vi "Get Head.vi"(11 "Snake in":refnum<class "Snake.lvclass">) -> (2 "Coordinates":T1)   [LabVIEW 2020, in "Snake.lvclass"]
uses:
  Snake.lvclass
  Type Defs/Coordinates.ctl
  Snake.lvclass/Snake.ctl
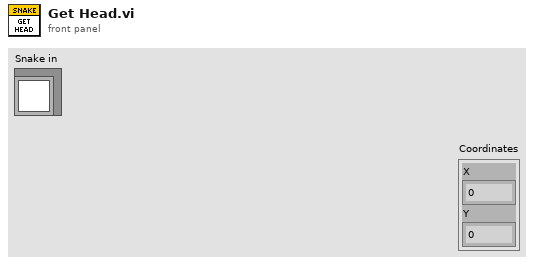
[diagram p1: front panel]
types:
  T1 = typedef "Coordinates.ctl" = cluster{"X":i32, "Y":i32}
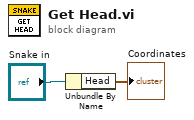
[diagram p0: block diagram]
diagram:
  n1 = Unbundle By Name("Snake in") -> ("Head"=→"Coordinates":T1)
